vi "Add String to Source.vi"(8 "Content":string=" and ", 9 "True/f":bool, 10 "Operation":enum16{"Read", "Write"}(ring)=enum."Write", 11 "Source":string) -> (3 "Result":string)   [LabVIEW 2015, in "ActorManagement.lvlib" / "UserInfoManageUI.lvclass"]
uses:
  UserInfoManageUI.lvclass
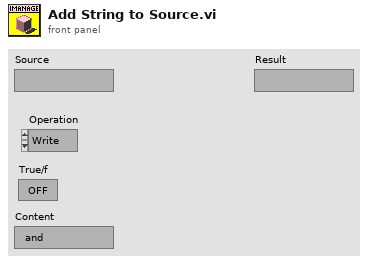
[diagram p1: front panel]
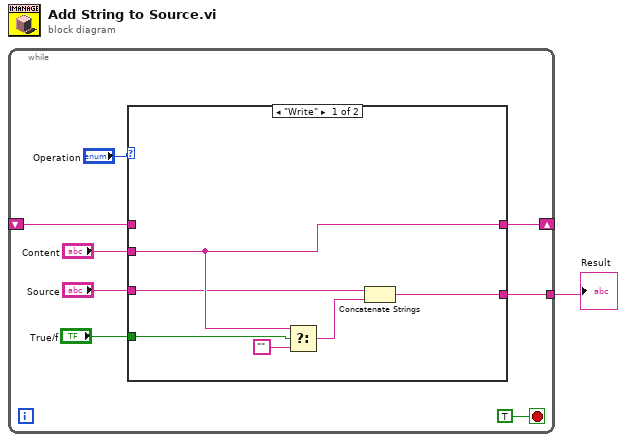
[diagram p0: block diagram]
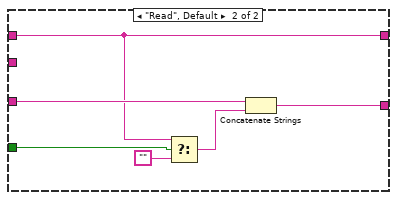
[diagram p2: hidden frame]
diagram:
  n1 = while {
    shift-right: [w5] -> _
    shift-left: _ -> [w4]
    tunnel: [w2] -> w1
    stop <- TRUE stop-if-true
    n2 = case shown="\"Write\"" "Operation" {
      tunnel: "Content" -> [w14 _]
      tunnel: "True/f" -> [w15 w21]
      tunnel: [w14 w16] -> w5
      tunnel: w4 -> [_ w16]
      tunnel: "Source" -> [w12 w19]
      tunnel: [w10 w17] -> w2
      frame "Write" {
        n3 = Select(t=w14, s=w15, f="") -> (s? t:f=w11:string)
        n4 = Concatenate Strings(w12, w11) -> (w10:string)
      }
      frame "Read", Default {
        n5 = Select(t=w16, s=w21, f="") -> (s? t:f=w18:string)
        n6 = Concatenate Strings(w19, w18) -> (w17:string)
      }
    }
  }
  "Result" <- w1
